vi "CheckGameBoardSearchLogic.vi"(7 "element":cluster{"row":i32, "col":i32}, 8 "error in (no error)":errorcluster, 9 "Current Color in":i32, 10 "Coloring Board in":cluster{"tile":T1, "color":i8}[][](array[cluster]), 11 "Queue in":refnum<queue>) -> (0 "error out":errorcluster, 1 "Current Color out":i32, 2 "Coloring Board out":cluster{"tile":T1, "color":i8}[][](array[cluster]), 3 "Queue out":refnum<queue>)   [LabVIEW 2020]
doc: "Somewhat bulky part of CheckGameBoard.vi\nExamines provided element.\nWall get -1, already colored element is skiped, uncolored element (0) is enqueued and a new color is prepared (+1)"
uses:
  TypeDef/tiles-key-trunct.ctl
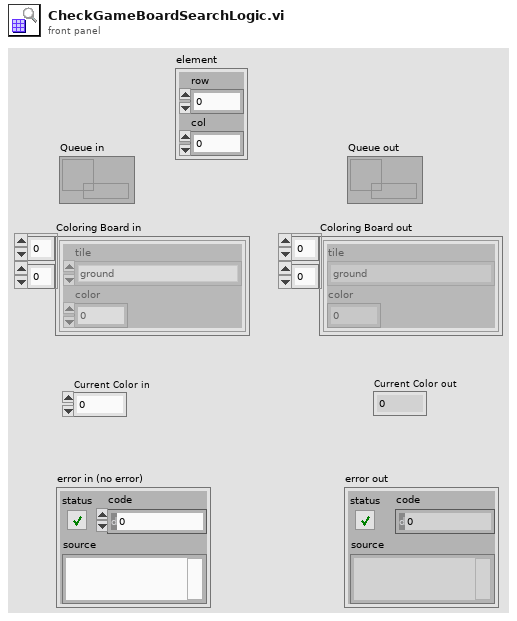
[diagram p1: front panel]
types:
  T1 = typedef "tiles-key-trunct.ctl" = enum16{"ground", "wall", "head (right)", "head (up)", "head (left)", "head (down)", "L-turn (right-up)", "L-turn (up-left)", "L-turn (left-down)", "L-turn (down-right)", "body (right)", "body (up)", "body (left)", "body (down)", "R-turn (right-down)", "R-turn (up-right)", "R-turn (left-up)", "R-turn (down-left)", "tail (right)", "tail (up)", "tail (left)", "tail (down)"}
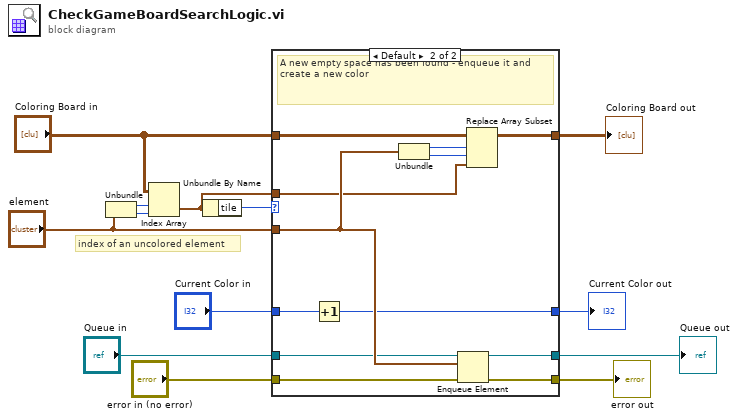
[diagram p0: block diagram]
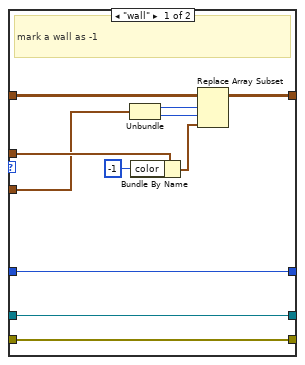
[diagram p2: hidden frame]
diagram:
  # "index of an uncolored element"
  n1 = Unbundle("element") -> ("row"=w3:i32, "col"=w4:i32)
  n2 = Index Array(array="Coloring Board in", index (row)=w3, index (col)=w4) -> (element=w6:cluster{"tile":T1, "color":i8})
  n3 = Unbundle By Name(w6) -> ("tile"=w5:T1)
  n4 = case shown="Default" w5 {
    tunnel: "error in (no error)" -> [w23 w29]
    tunnel: "Queue in" -> [w22 w28]
    tunnel: w6 -> [w24 w25]
    tunnel: [w23 w31] -> w7
    tunnel: [w22 w27] -> w8
    tunnel: "Coloring Board in" -> [w20 w36]
    tunnel: "element" -> [w17 w32]
    tunnel: [w19 w35] -> w10
    tunnel: "Current Color in" -> [w14 w30]
    tunnel: [w14 w26] -> w1
    frame "wall" {
      # "mark a wall as -1"
      n5 = Unbundle(w17) -> ("row"=w16:i32, "col"=w15:i32)
      n6 = Bundle By Name(cluster=w24, "color"=i8 -1) -> (w18:cluster{"tile":T1, "color":i8})
      n7 = Replace Array Subset(array=w20, new element=w18, index (row)=w16, index (col)=w15) -> (w19:cluster{"tile":T1, "color":i8}[][])
    }
    frame Default {
      # "A new empty space has been found - enqueue it and create a new color"
      n8 = Increment(x=w30) -> (x+1=w26:i32)
      n9 = Unbundle(w32) -> ("row"=w34:i32, "col"=w33:i32)
      n10 = Enqueue Element(queue=w28, element=w32, error in (no error)=w29) -> (queue out=w27:refnum<queue>, error out=w31:errorcluster)  [unwired: 1 in, 1 out]
      n11 = Replace Array Subset(array=w36, new element=w25, index (row)=w34, index (col)=w33) -> (w35:cluster{"tile":T1, "color":i8}[][])
    }
  }
  "Coloring Board out" <- w10
  "Queue out" <- w8
  "error out" <- w7
  "Current Color out" <- w1
